vi "UTEX Send.vi"(8 "error in":errorcluster, 10 "Changed Values?":T1, 11 "UT340 Controls":T2={"High Pass On"=FALSE, "High Pass Filter (MHz)"=1, "Low Pass On"=FALSE, "Low Pass Filter (MHz)"=20, "PE Gain (dB)"=1, "Voltage"=100, "Pulse Width (ns)"=2.0, "Mode"=FALSE, "PC Gain (dB)"=1, "Trig Source"=FALSE, "Rep Rate (Hz)"=0, "PULSE"=FALSE} {"Low Pass Filter (MHz)" min=20 step=1; "High Pass Filter (MHz)" min=1 max=20 step=1; "Pulse Width (ns)" min=2.0 max=71.75; "Voltage" min=100 max=250 step=2; "PC Gain (dB)" min=-6 max=60 step=1; "PE Gain (dB)" min=-6 max=60 step=1}) -> (0 "error out":errorcluster)   [LabVIEW 2022 SP3]
uses:
  Controls/UTEX Controls.ctl
  PulserGlobals.vi
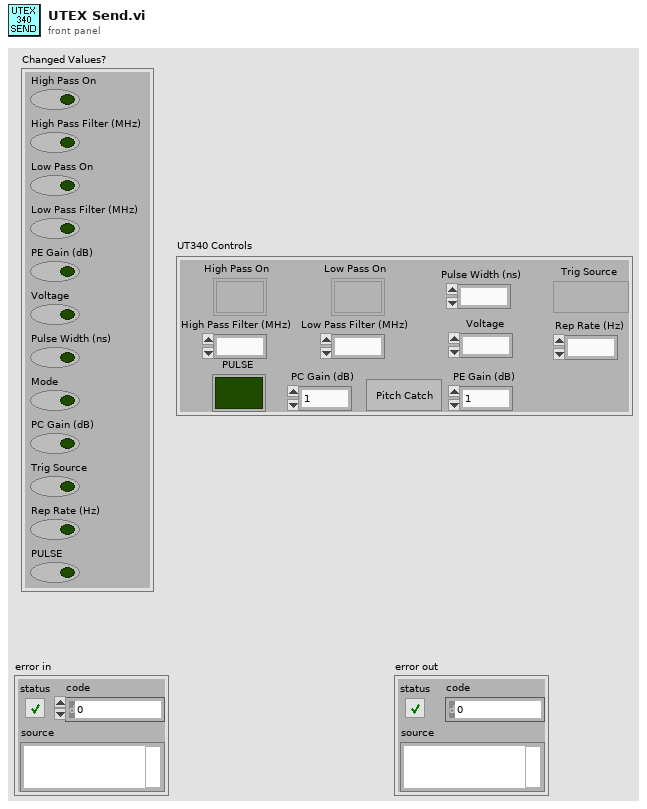
[diagram p1: front panel]
types:
  T1 = cluster{"High Pass On":bool, "High Pass Filter (MHz)":bool, "Low Pass On":bool, "Low Pass Filter (MHz)":bool, "PE Gain (dB)":bool, "Voltage":bool, "Pulse Width (ns)":bool, "Mode":bool, "PC Gain (dB)":bool, "Trig Source":bool, "Rep Rate (Hz)":bool, "PULSE":bool}
  T2 = typedef "UTEX Controls.ctl" = cluster{"High Pass On":bool, "High Pass Filter (MHz)":i16, "Low Pass On":bool, "Low Pass Filter (MHz)":i16, "PE Gain (dB)":i16, "Voltage":i16, "Pulse Width (ns)":dbl, "Mode":bool, "PC Gain (dB)":i16, "Trig Source":bool, "Rep Rate (Hz)":i16, "PULSE":bool}
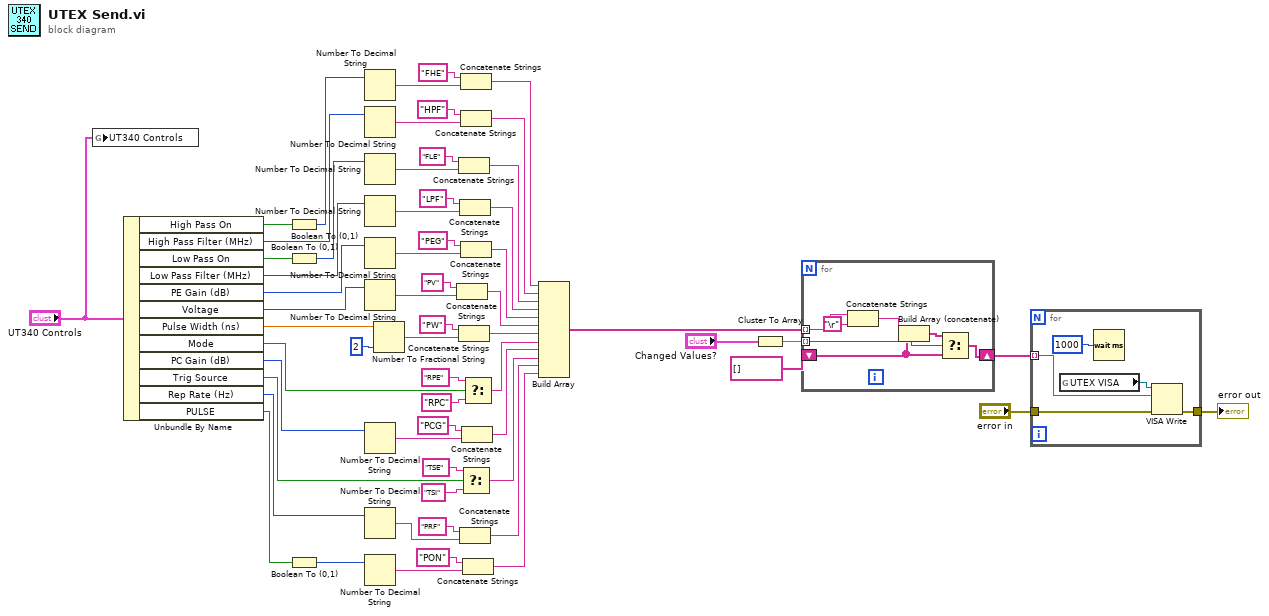
[diagram p0: block diagram]
diagram:
  n1 = global write "PulserGlobals.vi" "UT340 Controls"("UT340 Controls") -> ()
  n2 = Unbundle By Name("UT340 Controls") -> ("High Pass On"=w41:bool, "High Pass Filter (MHz)"=w54:i16, "Low Pass On"=w57:bool, "Low Pass Filter (MHz)"=w51:i16, "PE Gain (dB)"=w48:i16, "Voltage"=w45:i16, "Pulse Width (ns)"=w28:dbl, "Mode"=w19:bool, "PC Gain (dB)"=w32:i16, "Trig Source"=w22:bool, "Rep Rate (Hz)"=w25:i16, "PULSE"=w35:bool)
  n3 = Boolean To (0,1)(Boolean=w41) -> (0, 1=w44:i16)
  n4 = Boolean To (0,1)(Boolean=w57) -> (0, 1=w60:i16)
  n5 = Boolean To (0,1)(Boolean=w35) -> (0, 1=w38:i16)
  n6 = Number To Decimal String(number=w44) -> (decimal integer string=w43:string)  [unwired: 1 in]
  n7 = Number To Decimal String(number=w54) -> (decimal integer string=w56:string)  [unwired: 1 in]
  n8 = Number To Decimal String(number=w60) -> (decimal integer string=w59:string)  [unwired: 1 in]
  n9 = Number To Decimal String(number=w51) -> (decimal integer string=w53:string)  [unwired: 1 in]
  n10 = Number To Decimal String(number=w48) -> (decimal integer string=w50:string)  [unwired: 1 in]
  n11 = Number To Decimal String(number=w45) -> (decimal integer string=w47:string)  [unwired: 1 in]
  n12 = Number To Decimal String(number=w32) -> (decimal integer string=w34:string)  [unwired: 1 in]
  n13 = Number To Decimal String(number=w25) -> (decimal integer string=w27:string)  [unwired: 1 in]
  n14 = Number To Decimal String(number=w38) -> (decimal integer string=w37:string)  [unwired: 1 in]
  n15 = Number To Fractional String(number=w28, precision (6)=i16 2) -> (F-format string=w30:string)  [unwired: 2 in]
  n16 = Concatenate Strings("PV" ("string"), w47) -> (w8:string)
  n17 = Concatenate Strings("FLE" ("string"), w59) -> (w12:string)
  n18 = Concatenate Strings("PW" ("string"), w30) -> (w7:string)
  n19 = Concatenate Strings("LPF" ("string"), w53) -> (w10:string)
  n20 = Concatenate Strings("PRF" ("string"), w27) -> (w3:string)
  n21 = Concatenate Strings("FHE" ("string"), w43) -> (w14:string)
  n22 = Concatenate Strings("HPF" ("string"), w56) -> (w13:string)
  n23 = Concatenate Strings("PEG" ("string"), w50) -> (w9:string)
  n24 = Select(t="TSE" ("string"), s=w22, f="TSI") -> (s? t:f=w4:string)
  n25 = Concatenate Strings("PCG" ("string"), w34) -> (w5:string)
  n26 = Select(t="RPE" ("string"), s=w19, f="RPC") -> (s? t:f=w6:string)
  n27 = Concatenate Strings("PON" ("string"), w37) -> (w2:string)
  n28 = Build Array(w14, w13, w12, w10, w9, w8, w7, w6, w5, w4, w3, w2) -> (w11:string[])
  n29 = Cluster To Array(cluster="Changed Values?") -> (array=w18:bool[])
  n30 = for {
    tunnel: w18 -> [w67] mode=indexing
    shift-right: [w65] -> w15
    shift-left: string[] [] ("array") -> [w63]
    tunnel: w11 -> [w64] mode=indexing
    n31 = Concatenate Strings(w64, "\r") -> (w62:string)
    n32 = Build Array (concatenate)(w62, w63) -> (w66:string[])
    n33 = Select(t=w66, s=w67, f=w63) -> (s? t:f=w65:string[])
  }
  n34 = for {
    tunnel: w15 -> [w72] mode=indexing
    tunnel: [w70] -> w40
    tunnel: "error in" -> [w69]
    n35 = global read "PulserGlobals.vi" "UTEX VISA"() -> (w71:refnum<visa-resource-name>)
    n36 = Wait (ms)(milliseconds to wait=u32 1000) -> ()  [unwired: 1 out]
    n37 = VISA Write(VISA resource name=w71, write buffer=w72, error in (no error)=w69) -> (error out=w70:errorcluster)  [unwired: 2 out]
  }
  "error out" <- w40
